vi "H.Signal.vi"() -> (2 "element":bool, 4 "Slide servo home RS":bool, 6 "HI Bit Auto":bool, 8 "Error M Auto":string, 10 "Error Message":string, 15 "Bool_H Sig":bool)   [LabVIEW 2015]
uses:
  Galobal variable_TI.vi
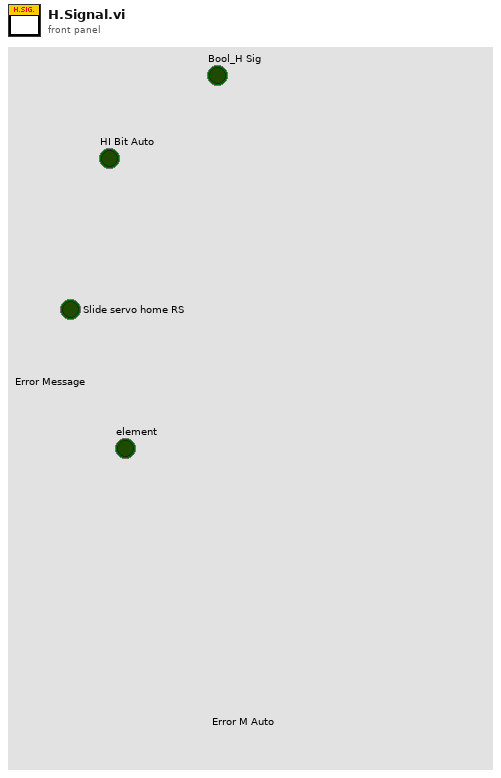
[diagram p1: front panel]
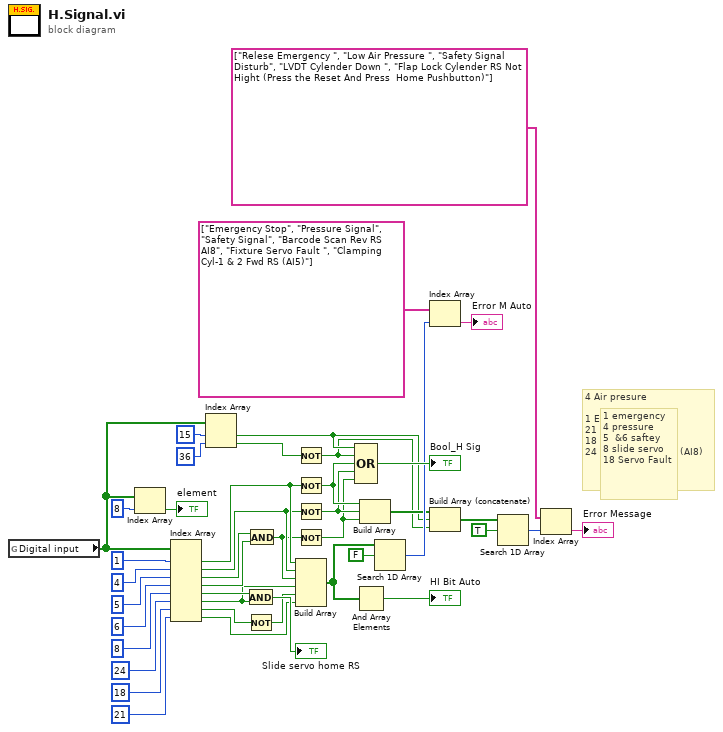
[diagram p0: block diagram]
diagram:
  # "4 Air presure\n  \n1 Emergency\n21 fixture clamp\n18 Servo Fault\n24 Bar code Rev RS (AI8)"
  # "1 emergency\n4 pressure\n5  &6 saftey\n8 slide servo\n18 Servo Fault"
  n1 = global read "Galobal variable_TI.vi" "Digital input"() -> (w8:bool[])
  n2 = Index Array(array=w8, index=8) -> (element=→"element":bool)
  n3 = Index Array(array=w8, index #1=1 ("index"), index #2=4 ("index"), index #3=5 ("index"), index #4=6 ("index"), index #5=8 ("index"), index #6=24 ("index"), index #7=18 ("index"), index #8=21 ("index")) -> (element #1=w25:bool, element #2=w24:bool, element #3=w38:bool, element #4=w37:bool, element #5=w27:bool, element #6=w22:bool, element #7=w16:bool, element #8=w12:bool)
  n4 = Index Array(array=w8, index #1=15 ("index"), index #2=36 ("index")) -> (element #1=w2:bool, element #2=w3:bool)
  n5 = And(x=w27, y=w22) -> (x .and. y?=→"Slide servo home RS":bool)
  n6 = Not(x=w16) -> (.not. x?=w11:bool)
  n7 = And(x=w38, y=w37) -> (x .and. y?=w23:bool)
  n8 = Not(x=w3) -> (.not. x?=w1:bool)
  n9 = Not(x=w25) -> (.not. x?=w31:bool)
  n10 = Not(x=w24) -> (.not. x?=w30:bool)
  n11 = Not(x=w23) -> (.not. x?=w29:bool)
  n12 = Build Array(w25, w24, w23, w22, w11, w12) -> (w15:bool[])
  n13 = Compound Arithmetic op=OR(w2, w1, w31, w30, w29) -> (→"Bool_H Sig":bool)
  n14 = And Array Elements(Boolean array=w15) -> (logical AND=→"HI Bit Auto":bool)
  n15 = Build Array(w31, w30, w29) -> (w6:bool[])
  n16 = Search 1D Array(1D array=w15, element=FALSE) -> (index of element=w20:i32)  [unwired: 1 in]
  n17 = Index Array(array=string[] ["Emergency Stop", "Pressure Signal", "Safety Signal", "Barcode Scan Rev RS AI8", "Fixture Servo Fault ", "Clamping Cyl-1 & 2 Fwd RS (AI5)"], index=w20) -> (element=→"Error M Auto":string)
  n18 = Build Array (concatenate)(w6, w2, w1) -> (w5:bool[])
  n19 = Search 1D Array(1D array=w5, element=TRUE) -> (index of element=w35:i32)  [unwired: 1 in]
  n20 = Index Array(array=string[] ["Relese Emergency ", "Low Air Pressure ", "Safety Signal Disturb", "LVDT Cylender Down ", "Flap Lock Cylender RS Not Hight (Press the Reset And Press  Home Pushbutton)"], index=w35) -> (element=→"Error Message":string)
